vi "UDP Named Service - Client.vi"() -> ()   [LabVIEW 2023]
doc: "This VI implements a client for the UDP Named Service - Server.vi. It connects to a service by specifying the server address and the name of the service. The client receives the string sent by the server, displays the string and closes the connection."
panel:
  out "Message from Server":string
  # "Overview: Demonstrates the use of the UDP functions to connect to a UDP server VI via named service and receive data.\nInstructions:\n1. Ensure UDP Named Service - Server.vi is already running.\n2. Run the VI."
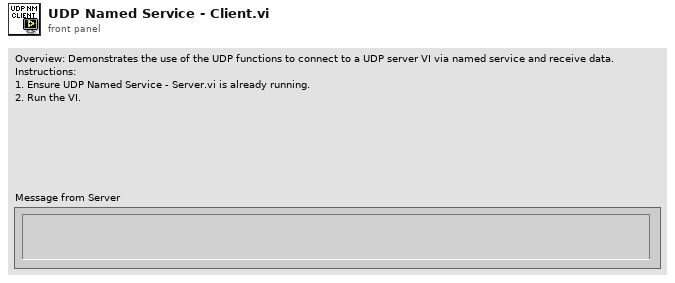
[diagram p1: front panel]
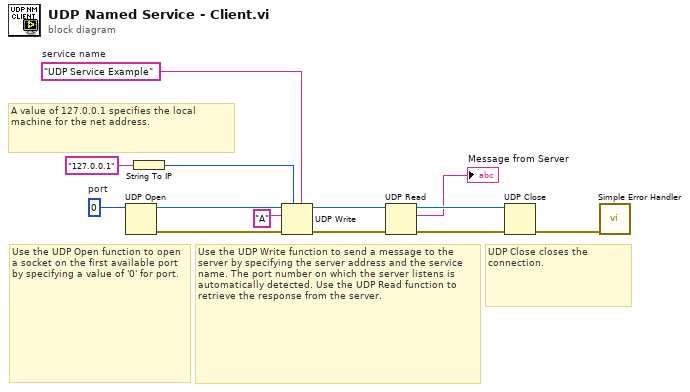
[diagram p0: block diagram]
diagram:
  w4 = "UDP Service Example"  # service name
  w10 = u16 0  # port
  # "UDP Close closes the connection."
  # "A value of 127.0.0.1 specifies the local machine for the net address."
  # "Use the UDP Open function to open a socket on the first available port by specifying a value of '0' for port."
  # "Use the UDP Write function to send a message to the server by specifying the server address and the service name. The port number on which the server listens is automatically detected. Use the UDP Read function to retrieve the response from the server."
  n1 = UDP Open(11:w10) -> (port=w12:refnum<k16>, 0:w13:errorcluster)  [unwired: 4 in, 1 out]
  n2 = String To IP(1:"127.0.0.1") -> (0:w8:u32)
  n3 = UDP Write(address=w8, port or service name=w4, connection ID=w12, data in="A", 8:w13) -> (error out=w7:errorcluster, 3:w6:refnum<k16>)  [unwired: 1 in]
  n4 = UDP Read(connection ID=w6, 8:w7) -> (data out=→"Message from Server":string, error out=w3:errorcluster, 3:w5:refnum<k16>)  [unwired: 2 in, 2 out]
  n5 = UDP Close(connection ID=w5, 8:w3) -> (error out=w11:errorcluster)  [unwired: 1 out]
  n6 = call <vilib>:"Simple Error Handler.vi"("error in (no error)"=w11) -> ()  [unwired: 4 in, 5 out]
